vi "Export DTC Control.vi"(8 "error in (no error)":errorcluster, 10 "GUID":string, 11 "Section Ref in":T4 format="%.0x") -> (0 "error out":errorcluster, 1 "Frame Settings Array":T1[](array[typedef]) {"Signals"."Byte Order" items=["Little Endian", "Big Endian"]; "Signals"."Data Type" items=["Signed", "Unsigned", "IEEE Float"]}, 2 "Frame Refs":T5[](array[typedef]) {"Signal Refs" format="%.0x"}, 3 "Section Ref out":T4 format="%.0x")   [LabVIEW 2015, in "Diagnostics Addon System Explorer.lvlib"]
uses:
  Diagnostics Addon System Explorer.lvlib
  <vilib>/NI Veristand/Custom Device API/Custom Device Item Ref.ctl
  Types/Frame Signal VS References.ctl
  Shared/Types/Common Frame Parameters.ctl
  Shared/Types/MessageType Selector.ctl
  Shared/Types/Signal Parameters.ctl
  Types/FG Action.ctl
  Signal Parameters FG.vi
  <vilib>/NI Veristand/Custom Device API/NI VeriStand - Get Custom Device Channel Data.vi
  <vilib>/NI Veristand/Custom Device API/NI VeriStand - Get Item Description.vi
  <vilib>/NI Veristand/Custom Device API/NI VeriStand - Get Item Property.vi
  <vilib>/NI Veristand/Custom Device API/Get Item Property (String).vi
  <vilib>/NI Veristand/Custom Device API/Get Item Property (Double).vi
  <vilib>/NI Veristand/Custom Device API/Get Item Property (U32).vi
  <vilib>/NI Veristand/Custom Device API/NI VeriStand - Set Item Property.vi
  <vilib>/NI Veristand/Custom Device API/Set Item Property (String).vi
  <vilib>/NI Veristand/Custom Device API/Set Item Property (Double).vi
  <vilib>/NI Veristand/Custom Device API/Set Item Property (U32).vi
  Shared/SubVIs/GUID Lookup.vi
  <vilib>/NI Veristand/Custom Device API/NI VeriStand - Get Item Children.vi
  <vilib>/NI Veristand/Custom Device Tools/Custom Device Utility Library/NI VeriStand - Search for Item by GUID.vi
  <vilib>/NI Veristand/Custom Device Tools/Custom Device Utility Library/Custom Device Utility Library.lvlib
  <vilib>/NI Veristand/Custom Device API/Custom Device API.lvlib
  Shared/Diagnostics Addon Shared.lvlib
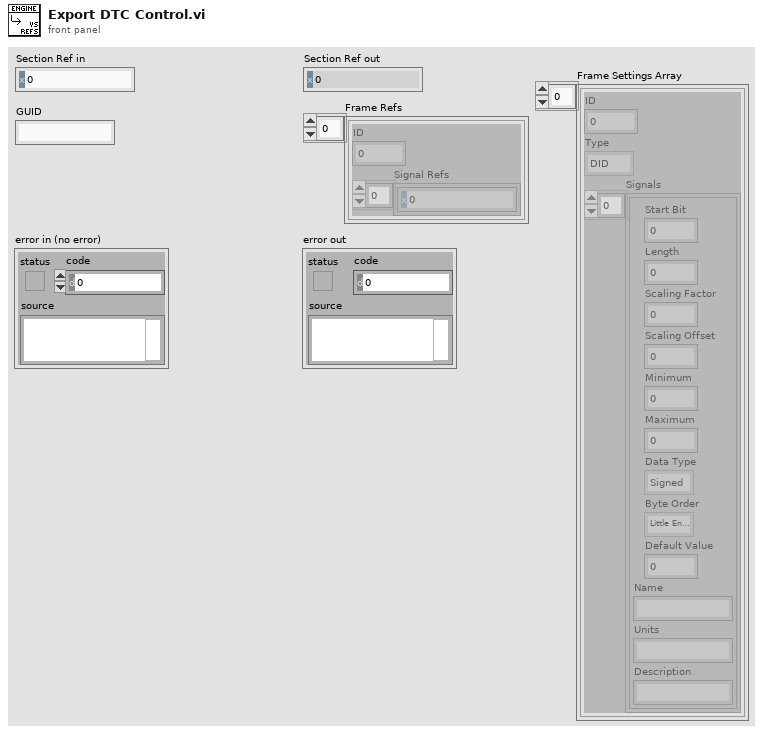
[diagram p1: front panel]
types:
  T1 = typedef "Diagnostics Addon Shared.lvlib/Common Frame Parameters.ctl" = cluster{"ID":u32, "Type":T2, "Signals":T3[]}
  T2 = typedef "Diagnostics Addon Shared.lvlib/MessageType Selector.ctl" = enum16{"DID", "PID", "CPID", "Write Memory", "Read Memory", "DTC Control", "IO Cmd", "IO Resp", "Routine Start Cmd", "Routine Start Resp", "Routine Status Cmd", "Routine Status Resp", "Routine Stop Cmd", "Routine Stop Resp"}
  T3 = typedef "Diagnostics Addon Shared.lvlib/Signal Parameters.ctl" = cluster{"Start Bit":u8, "Length":u8, "Scaling Factor":dbl, "Scaling Offset":dbl, "Minimum":dbl, "Maximum":dbl, "Data Type":u32, "Byte Order":u32, "Default Value":dbl, "Name":string, "Units":string, "Description":string}
  T4 = typedef "Custom Device API.lvlib/Custom Device Item Ref.ctl" = u64
  T5 = typedef "Diagnostics Addon System Explorer.lvlib/Frame Signal VS References.ctl" = cluster{"ID":u32, "Signal Refs":T4[]}
  T6 = typedef "Diagnostics Addon System Explorer.lvlib/FG Action.ctl" = enum16{"Get", "Set"}
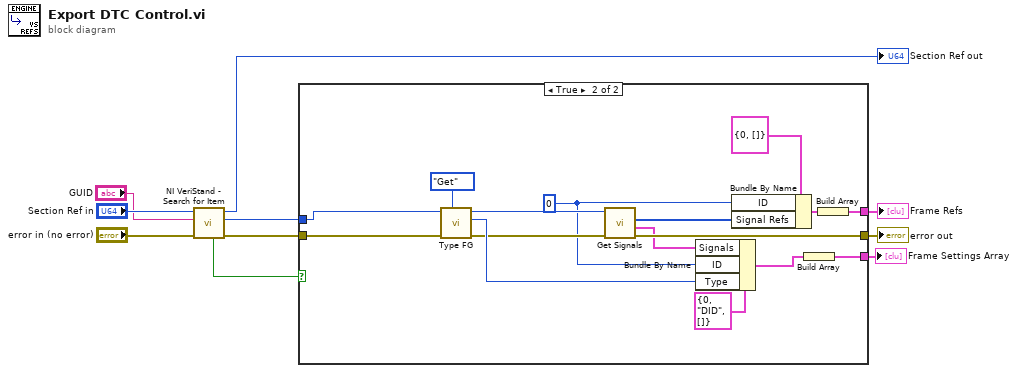
[diagram p0: block diagram]
diagram:
  n1 = call-poly <vilib>:"NI VeriStand - Search for Item.vi"("error in"="error in (no error)", "Item GUID"="GUID", "Section Ref in"="Section Ref in") -> ("error out"=w4:errorcluster, "Item Ref"=w5:T4, "Section Ref out"=→"Section Ref out":T4, "Found"=w2:bool)  [unwired: 5 in]
  n2 = case shown="True" w2 {
    tunnel: [w11 w27] -> w9
    tunnel: [_ w13] -> w8
    tunnel: w5 -> [_ w17]
    tunnel: w4 -> [w11 w24]
    tunnel: [_ w12] -> w1
    frame False {
    }
    frame True {
      w14 = 0
      n3 = call "Type FG.vi"("Action"=FG_Action."Get", "error in (no error)"=w24, "Device Item Ref in"=w17) -> ("error out"=w16:errorcluster, "Type"=w18:T2, "Device Item Ref out"=w15:T4)  [unwired: 6 in]
      n4 = call "Get Signals.vi"("error in (no error)"=w16, "Device Item Ref out"=w15) -> ("error out"=w27:errorcluster, "Parameters"=w20:T3[], "Child Refs"=w22:T4[])  [unwired: 6 in, 1 out]
      n5 = Bundle By Name(cluster=T1 {"ID"=0, "Type"=enum."DID", "Signals"=[]} ("PID In"), "Signals"=w20, "ID"=w14, "Type"=w18) -> (w25:T1)
      n6 = Bundle By Name(cluster=T5 {"ID"=0, "Signal Refs"=[]}, "ID"=w14, "Signal Refs"=w22) -> (w26:T5)
      n7 = Build Array(w25) -> (w12:T1[])
      n8 = Build Array(w26) -> (w13:T5[])
    }
  }
  "error out" <- w9
  "Frame Refs" <- w8
  "Frame Settings Array" <- w1
